vi "Generate jpg.vi"() -> ()   [LabVIEW 2020]
uses:
  <vilib>/vision/Image Controls.llb/IMAQ Image.ctl
  <vilib>/vision/NI_Vision_Development_Module.lvlib
panel:
  in  "minimum":dbl
  in  "maximum":dbl
  in  "Resolution":i32=512
  out "Background out":T1
  out "error out":errorcluster
  in  "error in (no error)":errorcluster
  in  "Page":i32=1
  in  "Image File Path":path=path "E:/Users/Anil/SA02836H.20160226/LAOSTO0004.ibw"
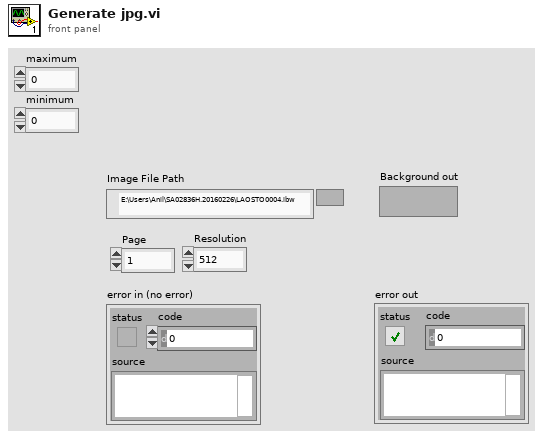
[diagram p1: front panel]
types:
  T1 = typedef "IMAQ Image.ctl" = refnum<image>
  T2 = typedef "Image Type" = u32
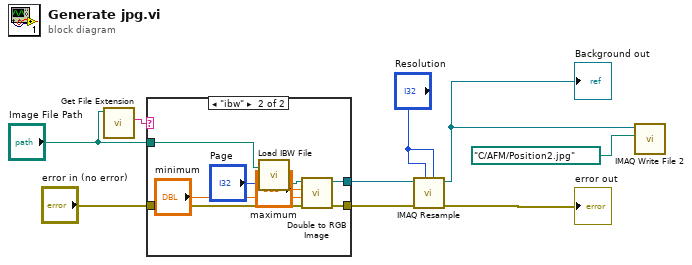
[diagram p0: block diagram]
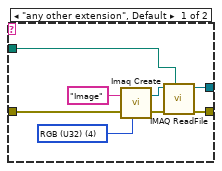
[diagram p2: hidden frame]
diagram:
  n1 = call <vilib>:"Get File Extension.vi"("file"="Image File Path") -> ("lowercase file extension"=w7:string)  [unwired: 6 in, 4 out]
  n2 = case shown="\"ibw\"" w7 {
    tunnel: [w17 w22] -> w6
    tunnel: [w16 w23] -> w5
    tunnel: "Image File Path" -> [w15 w25]
    tunnel: "error in (no error)" -> [w10 w20]
    frame "any other extension", Default {
      w14 = T2 4 items=["Grayscale (U8)", "Grayscale (I16)", "Grayscale (SGL)", "Complex (CSG)", "RGB (U32)", "HSL (U32)", "RGB (U64)", "Grayscale (U16)"] ("Image Type")
      n3 = call "Imaq Create"("Image Name"="Image", "Image Type"=w14, "error in (no error)"=w10) -> ("New Image"=w11:T1, "error out"=w12:errorcluster)  [unwired: 2 in]
      n4 = call "IMAQ ReadFile"("File Path"=w15, "error in (no error)"=w12, "Image"=w11) -> ("error out"=w16:errorcluster, "Image Out"=w17:T1)  [unwired: 4 in, 3 out]
    }
    frame "ibw" {
      n5 = call "Load IBW File.vi"("Page"="Page", "file path (dialog if empty)"=w25) -> ("Image"=w21:T1)  [unwired: 1 out]
      n6 = call "Double to RGB Image.vi"("error in (no error)"=w20, "minimum"="minimum", "maximum"="maximum", "Image Reference In"=w21) -> ("error out"=w23:errorcluster, "Image Reference Out"=w22:T1)  [unwired: 6 in]
    }
  }
  n7 = call "IMAQ Resample"("X Resolution"="Resolution", "Y Resolution"="Resolution", "error in (no error)"=w5, "Image Src"=w6) -> ("error out"=→"error out":errorcluster, "Image Dst Out"=w1:T1)  [unwired: 6 in]
  "Background out" <- w1
  n8 = call-poly "IMAQ Write File 2"("File Path"=path "C:/AFM/Position2.jpg", "Image"=w1) -> ()  [unwired: 8 in, 2 out]
